vi "LVClient2011.vi"() -> ()   [LabVIEW 2015]
panel:
  out "Error":string
  in  "address":string="localhost"
  in  "remote port or service name":u16=7000
  out "String":string
  out "data lenl":i32
  in  "Stop Server":bool
  in  "Stop Client":bool
  in  "Init Button":bool
  in  "Play Button":bool
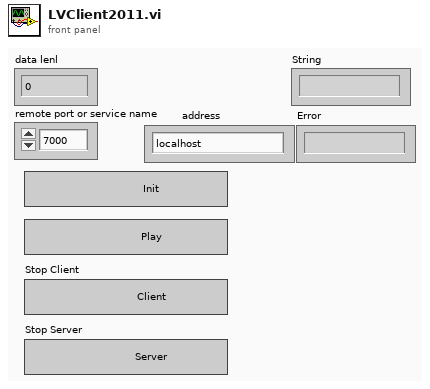
[diagram p1: front panel]
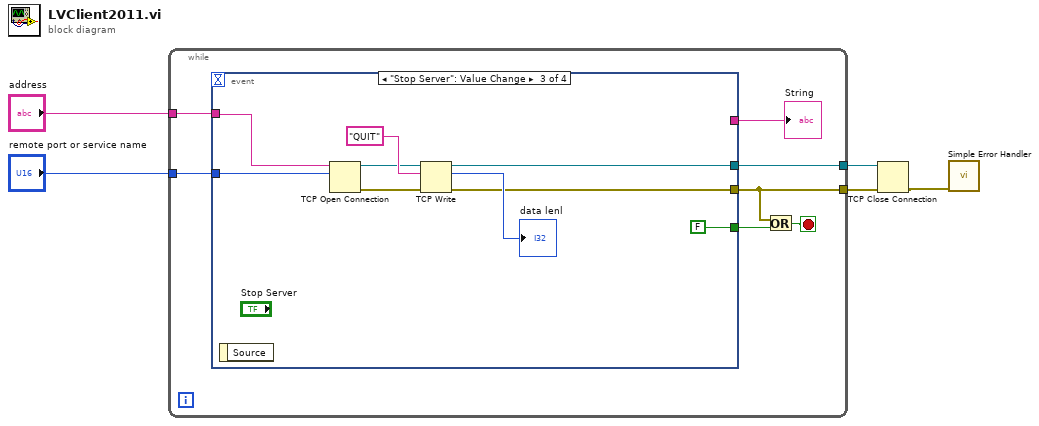
[diagram p0: block diagram]
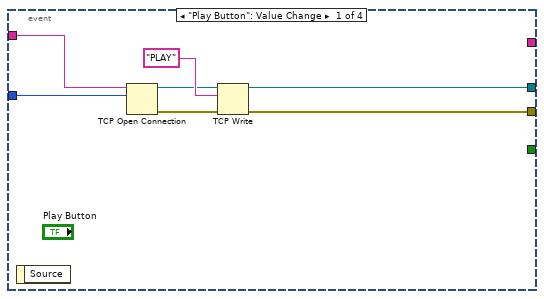
[diagram p2: hidden frame]
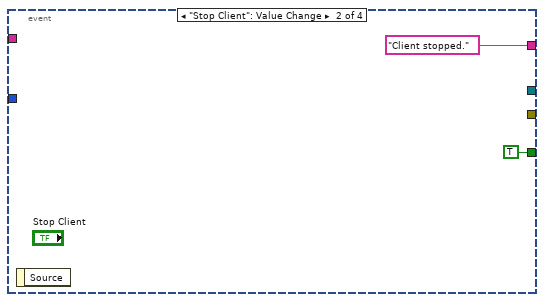
[diagram p3: hidden frame]
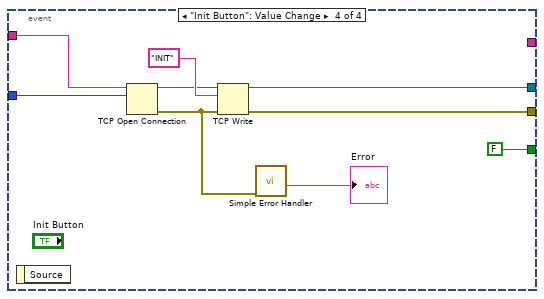
[diagram p4: hidden frame]
diagram:
  n1 = while {
    tunnel: [w12] -> w2
    tunnel: "remote port or service name" -> [w7]
    tunnel: "address" -> [w8]
    tunnel: [w6] -> w3
    stop <- w11 stop-if-true
    n2 = event shown="[2] \"Stop Server\": Value Change" {
      selector: _ -> [_ _ _ _]
      dyn-events: _ -> [_ _ _ _]
      timeout: _ -> [_ _ _ _]
      tunnel: [w13 _ w23 w34] -> w12
      tunnel: [_ TRUE FALSE FALSE] -> w10
      tunnel: [_ "Client stopped." ("data out") _ _] -> w9
      tunnel: w8 -> [w16 _ w24 w35]
      tunnel: w7 -> [w15 _ w25 w36]
      tunnel: [w14 _ w22 w33] -> w6
      event "Play Button": Value Change {
        n3 = event-data() -> ()  [unwired: 1 in, 1 out]
        n4 = TCP Open Connection(address=w16, remote port or service name=w15) -> (connection ID=w18:refnum<k5>, error out=w17:errorcluster)  [unwired: 3 in]
        n5 = TCP Write(connection ID=w18, data in="PLAY", error in (no error)=w17) -> (connection ID out=w14:refnum<k5>, error out=w13:errorcluster)  [unwired: 1 in, 1 out]
      }
      event "Stop Client": Value Change {
        n6 = event-data() -> ()  [unwired: 1 in, 1 out]
      }
      event "Stop Server": Value Change {
        n7 = event-data() -> ()  [unwired: 1 in, 1 out]
        n8 = TCP Open Connection(address=w24, remote port or service name=w25) -> (connection ID=w29:refnum<k5>, error out=w28:errorcluster)  [unwired: 3 in]
        n9 = TCP Write(connection ID=w29, data in="QUIT", error in (no error)=w28) -> (connection ID out=w22:refnum<k5>, bytes written=→"data lenl":i32, error out=w23:errorcluster)  [unwired: 1 in]
      }
      event "Init Button": Value Change {
        n10 = event-data() -> ()  [unwired: 1 in, 1 out]
        n11 = TCP Open Connection(address=w35, remote port or service name=w36) -> (connection ID=w38:refnum<k5>, error out=w32:errorcluster)  [unwired: 3 in]
        n12 = TCP Write(connection ID=w38, data in="INIT", error in (no error)=w32) -> (connection ID out=w33:refnum<k5>, error out=w34:errorcluster)  [unwired: 1 in, 1 out]
        n13 = call <vilib>:"Simple Error Handler.vi"("error in (no error)"=w32) -> ("source out"=→"Error":string)  [unwired: 4 in, 4 out]
      }
    }
    "String" <- w9
    n14 = Or(x=w12, y=w10) -> (x .or. y?=w11:bool)
  }
  n15 = TCP Close Connection(connection ID=w3, error in (no error)=w2) -> (error out=w1:errorcluster)  [unwired: 1 in, 1 out]
  n16 = call <vilib>:"Simple Error Handler.vi"("error in (no error)"=w1) -> ()  [unwired: 4 in, 5 out]
